vi "Initialize phase.vi"(8 "error in (no error)":errorcluster, 11 "Programming Logicv2 in":refnum<class "Programming Logicv2.lvclass">) -> (0 "error out":errorcluster, 3 "Programming Logicv2 out":refnum<class "Programming Logicv2.lvclass">)   [LabVIEW 2014, in "Main Libraryv2.lvlib" / "Programming Logicv2.lvclass"]
uses:
  Programming Logicv2.lvclass
  <vilib>/NI/Modbus Library/API/Wrapper/API Main.lvlib
  <vilib>/NI/Modbus Library/API/Wrapper/Create Serial Master.vi
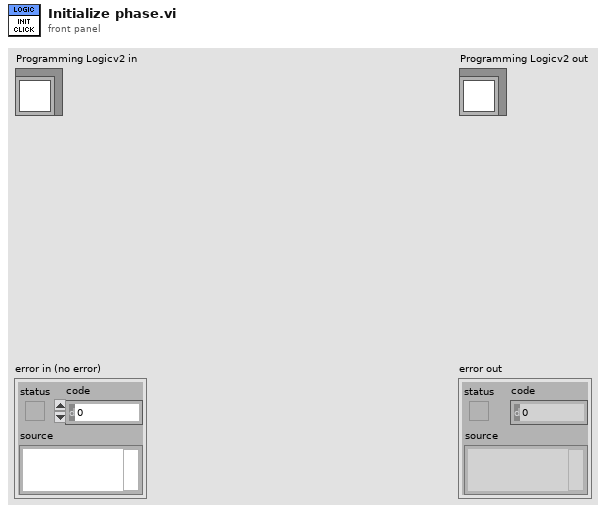
[diagram p1: front panel]
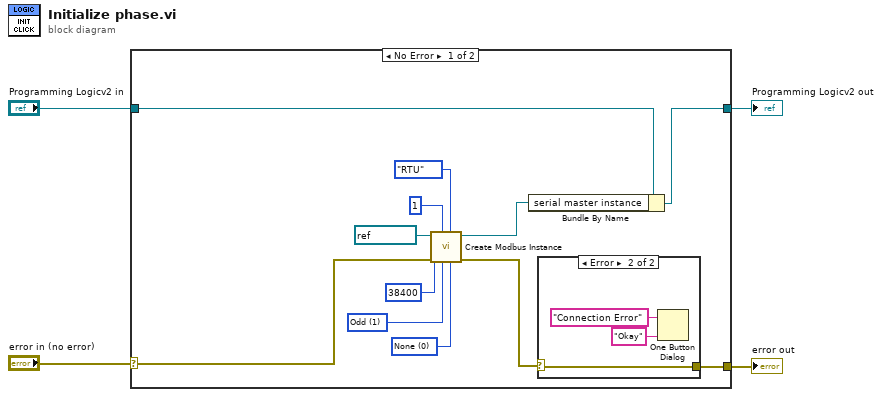
[diagram p0: block diagram]
diagram:
  n1 = case shown="No Error" "error in (no error)" {
    selector: "error in (no error)" -> [w7 w22]
    tunnel: [w8 w22] -> w3
    tunnel: [w6 w21] -> w1
    tunnel: "Programming Logicv2 in" -> [w5 w21]
    frame No Error {
      w14 = u16 0 items=["None", "XON/XOFF", "RTS/CTS", "XON/XOFF & RTS/CTS", "DTR/DSR", "XON/XOFF & DTR/DSR"] ("flow control (none)")
      w15 = u16 1 items=["None", "Odd", "Even", "Mark", "Space"] ("parity (even)")
      n2 = call-poly <vilib>:"Create Modbus Instance.vi"("flow control (none)"=w14, "serial type"=enum16{"RTU", "ASCII"}."RTU", "parity (even)"=w15, "unit ID"=u8 1, "error in"=w7, "baud rate"=u32 38400, "VISA resource name"=refnum<visa-resource-name> "COM1") -> ("error out"=w9:errorcluster, "serial master instance"=w11:refnum<class "Modbus Master.lvclass">)  [unwired: 3 in]
      n3 = Bundle By Name(cluster=w5, "serial master instance"=w11) -> (w6:refnum<class "Programming Logicv2.lvclass">)
      n4 = case shown="Error" w9 {
        selector: w9 -> [w17 w20]
        tunnel: [w17 w20] -> w8
        frame No Error {
        }
        frame Error {
          n5 = One Button Dialog(message="Connection Error", button name ("OK")="Okay") -> ()  [unwired: 1 out]
        }
      }
    }
    frame Error {
    }
  }
  "error out" <- w3
  "Programming Logicv2 out" <- w1
